vi "Query Marker.vi"(8 "error in (no error)":errorcluster, 10 "Marker Number":u8=1, 11 "VNA-Keysight PNA in":refnum<class "VNA-Keysight PNA.lvclass">) -> (0 "error out":errorcluster, 1 "Data":dbl, 2 "Frequency":dbl, 3 "VNA-Keysight PNA out":refnum<class "VNA-Keysight PNA.lvclass">)   [LabVIEW 2020, in "VNA-Keysight PNA.lvclass"]
doc: "Query the marker on the active trace"
uses:
  VNA-Keysight PNA.lvclass
  C:/Sandbox/RF Bench/Source Code/WiSpry Test Framework/Instruments/Instrument.lvclass
  Instrument.lvclass/Instrument.ctl
  Instrument.lvclass
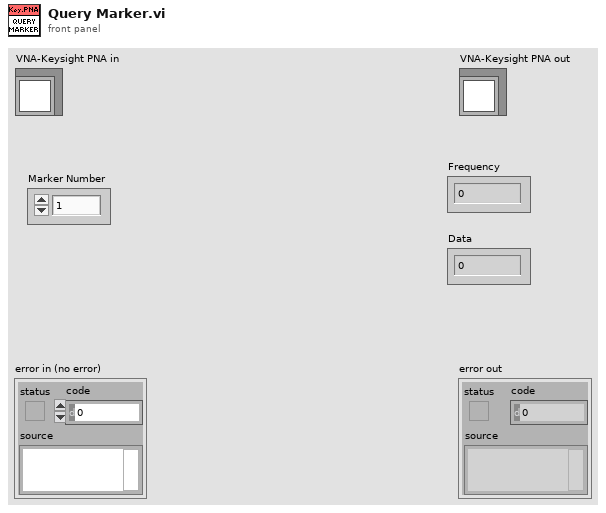
[diagram p1: front panel]
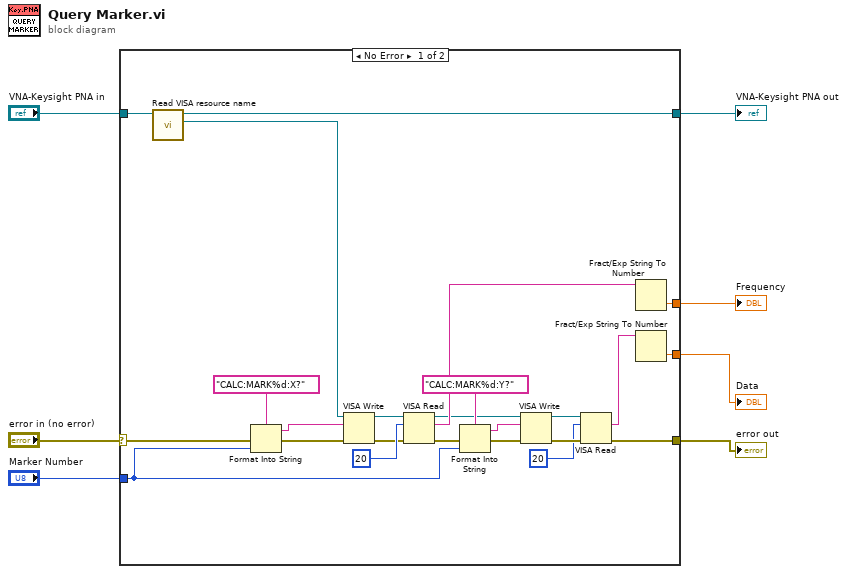
[diagram p0: block diagram]
diagram:
  n1 = case shown="No Error" "error in (no error)" {
    selector: "error in (no error)" -> [w17 w32]
    tunnel: [w30 w33] -> w6
    tunnel: "VNA-Keysight PNA in" -> [w31 w33]
    tunnel: [w14 w32] -> w7
    tunnel: "Marker Number" -> [w16 _]
    tunnel: [w12 _] -> w2
    tunnel: [w8 _] -> w1
    frame No Error {
      n2 = call "Read VISA resource name.vi"("Instrument in"=w31) -> ("VISA resource name"=w9:refnum<visa-resource-name>, "Instrument out"=w30:refnum<class "VNA-Keysight PNA.lvclass">)  [unwired: 9 in]
      n3 = Format Into String(format string="CALC:MARK%d:X?" ("write buffer"), error in=w17, w16) -> (resulting string=w19:string, error out=w20:errorcluster)  [unwired: 1 in]
      n4 = VISA Write(VISA resource name=w9, write buffer=w19, error in (no error)=w20) -> (VISA resource name out=w23:refnum<visa-resource-name>, error out=w21:errorcluster)  [unwired: 1 out]
      n5 = VISA Read(VISA resource name=w23, byte count=u32 20, error in (no error)=w21) -> (VISA resource name out=w10:refnum<visa-resource-name>, read buffer=w11:string, error out=w15:errorcluster)  [unwired: 1 out]
      n6 = Format Into String(format string="CALC:MARK%d:Y?" ("write buffer"), error in=w15, w16) -> (resulting string=w28:string, error out=w27:errorcluster)  [unwired: 1 in]
      n7 = VISA Write(VISA resource name=w10, write buffer=w28, error in (no error)=w27) -> (VISA resource name out=w24:refnum<visa-resource-name>, error out=w26:errorcluster)  [unwired: 1 out]
      n8 = VISA Read(VISA resource name=w24, byte count=u32 20, error in (no error)=w26) -> (read buffer=w13:string, error out=w14:errorcluster)  [unwired: 2 out]
      n9 = Fract/Exp String To Number(string=w11) -> (number=w8:dbl)  [unwired: 3 in, 1 out]
      n10 = Fract/Exp String To Number(string=w13) -> (number=w12:dbl)  [unwired: 3 in, 1 out]
    }
    frame Error {
    }
  }
  "error out" <- w7
  "VNA-Keysight PNA out" <- w6
  "Data" <- w2
  "Frequency" <- w1
